vi "StartSequenceAcquisition.vi"(8 "error in (no error)":errorcluster, 10 "DataExchange":T1, 11 "Camera_Prime95B in":refnum<class "Camera_Prime95B.lvclass">) -> (0 "error out":errorcluster, 3 "Camera_Prime95B out":refnum<class "Camera_Prime95B.lvclass">)   [LabVIEW 2020, in "Camera_Prime95B.lvlib" / "Camera_Prime95B.lvclass"]
uses:
  Camera_Prime95B.lvclass
  Hardware Abstraction Layer/Component/Device/Device/DataExchange.ctl
  Controls/AcquisitionParams.ctl
  Controls/Camera Status.ctl
  Camera_Prime95B.lvclass/Camera_Prime95B.ctl
  Hardware Abstraction Layer/Component/Device/Device/DeviceStatus.ctl
  Controls/Wait For Stop Status.ctl
  E:/Development/DevHardSoftware/MicroscopyFramework/Model/Hardware Layer/Real Hardware/Camera_Prime95B/Camera_Prime95B/Dependencies/PVCamNET.dll
  Dependencies/PVCamNET.dll
  Hardware Abstraction Layer/Component/Device/Device/Device.lvlib
  Interface/DataListener/DataListener.lvclass
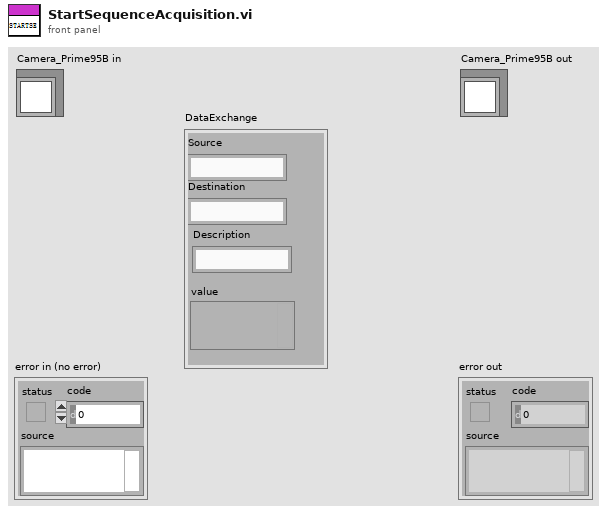
[diagram p1: front panel]
types:
  T1 = typedef "DataListener.lvclass/DataExchange.ctl" = cluster{"Source":string, "Destination":string, "Description":string, "value":variant}
  T2 = typedef "Camera_Prime95B.lvlib/Camera_Prime95B.lvclass/AcquisitionParams.ctl" = cluster{"Acq Mode":T3, "Save Path":path, "Stream Save Path":path, "SingleStack?":bool, "StreamToDisk?":bool, "Alert when finish?":bool}
  T3 = typedef "Camera_Prime95B.lvlib/Camera_Prime95B.lvclass/Camera Status.ctl" = i32
  T4 = typedef "Device.lvlib/DeviceStatus.ctl" = i32
  T5 = typedef "Camera_Prime95B.lvlib/Camera_Prime95B.lvclass/Wait For Stop Status.ctl" = i32
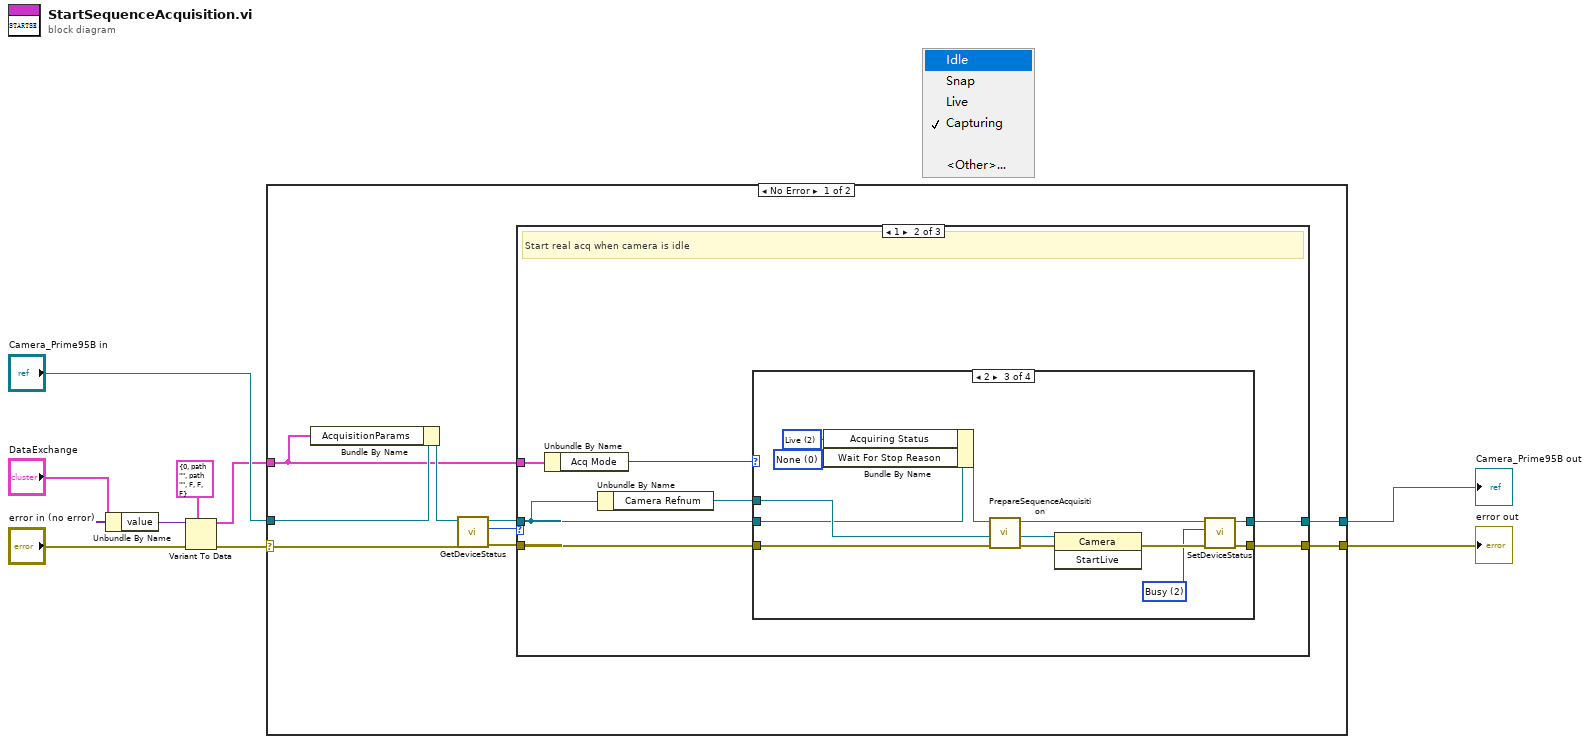
[diagram p0: block diagram]
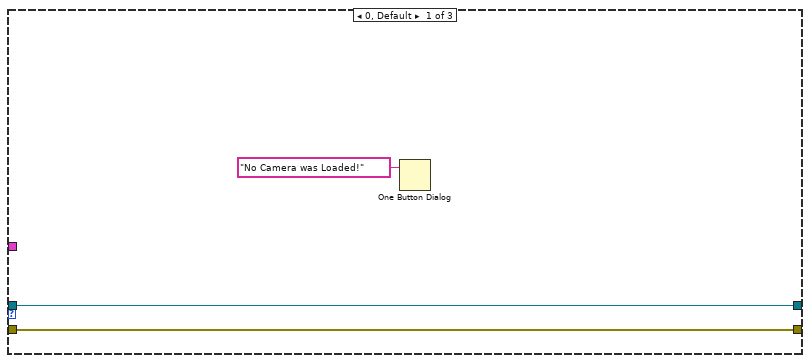
[diagram p2: hidden frame]
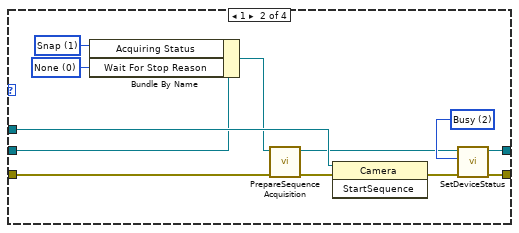
[diagram p4: hidden frame]
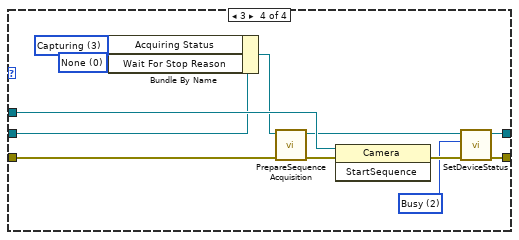
[diagram p5: hidden frame]
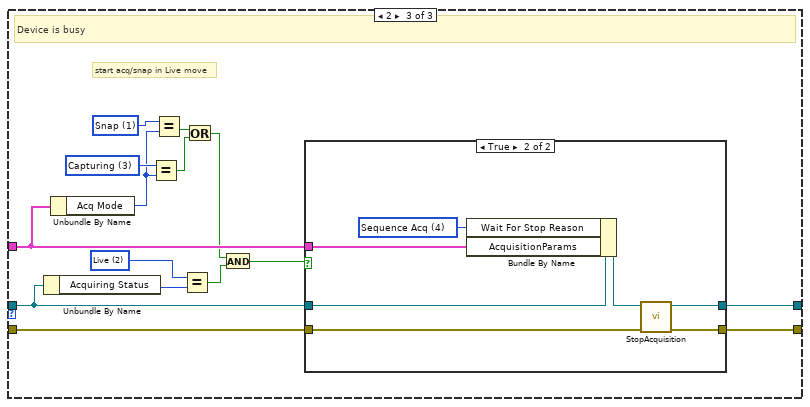
[diagram p6: hidden frame]
diagram:
  n1 = Unbundle By Name("DataExchange") -> ("value"=w5:variant)
  n2 = Variant To Data(error in="error in (no error)", type=T2 {"Acq Mode"=0, "Save Path"=path "", "Stream Save Path"=path "", "SingleStack?"=FALSE, "StreamToDisk?"=FALSE, "Alert when finish?"=FALSE} ("Acquisition Params"), Variant=w5) -> (data=w3:T2, error out=w2:errorcluster)
  n3 = case shown="No Error" w2 {
    selector: w2 -> [w18 w92]
    tunnel: [w15 w92] -> w6
    tunnel: "Camera_Prime95B in" -> [w17 w91]
    tunnel: [w16 w91] -> w7
    tunnel: w3 -> [w10 _]
    frame No Error {
      n4 = Bundle By Name(cluster=w17, "AcquisitionParams"=w10) -> (w11:refnum<class "Camera_Prime95B.lvclass">)
      n5 = call-dynamic "GetDeviceStatus.vi"("error in (no error)"=w18, "Camera_Prime95B in"=w11) -> ("error out"=w13:errorcluster, "Status"=w12:T4, "Camera_Prime95B out"=w14:refnum<class "Camera_Prime95B.lvclass">)  [unwired: 7 in]
      n6 = case shown="1" w12 {
        tunnel: w14 -> [w21 w23 w81]
        tunnel: [w21 w25 w80] -> w16
        tunnel: [w20 w28 w78] -> w15
        tunnel: w13 -> [w20 w26 w79]
        tunnel: w10 -> [_ w24 w77]
        frame 0, Default {
          n7 = One Button Dialog(message="No Camera was Loaded!") -> ()  [unwired: 1 in, 1 out]
        }
        frame 1 {
          # "Start real acq when camera is idle"
          n8 = Unbundle By Name(w24) -> ("Acq Mode"=w22:T3)
          n9 = Unbundle By Name(w23) -> ("Camera Refnum"=w27:refnum<k24>)
          n10 = case shown="2" w22 {
            tunnel: [w29 w39 w51 w63] -> w28
            tunnel: w26 -> [w29 w40 w52 w64]
            tunnel: w27 -> [_ w41 w53 w65]
            tunnel: w23 -> [w30 w32 w48 w57]
            tunnel: [w30 w38 w50 w62] -> w25
            frame 0, Default {
            }
            frame 1 {
              w34 = T3 1 items=["Idle", "Snap", "Live", "Capturing", ""] ("Acquiring Status")
              w35 = T5 0 items=["None", "Set Exposure", "Set Binning", "Set ROI", "Sequence Acq", ""] ("Wait For Stop Reason")
              w37 = T4 2 items=["Offline", "Idle", "Busy"] ("Status")
              n11 = Bundle By Name(cluster=w32, "Acquiring Status"=w34, "Wait For Stop Reason"=w35) -> (w31:refnum<class "Camera_Prime95B.lvclass">)
              n12 = call-dynamic "PrepareSequenceAcquisition.vi"("error in (no error)"=w40, "Camera_Prime95B in"=w31) -> ("error out"=w36:errorcluster, "Camera_Prime95B out"=w33:refnum<class "Camera_Prime95B.lvclass">)  [unwired: 8 in]
              n13 = invoke class="Camera" method="StartSequence"(reference=w41, error in=w36) -> (error out=w42:errorcluster)  [unwired: 1 in, 2 out]
              n14 = call-dynamic "SetDeviceStatus.vi"("error in (no error)"=w42, "Status"=w37, "Device in"=w33) -> ("error out"=w39:errorcluster, "Device out"=w38:refnum<class "Camera_Prime95B.lvclass">)  [unwired: 7 in]
            }
            frame 2 {
              w46 = T5 0 items=["None", "Set Exposure", "Set Binning", "Set ROI", "Sequence Acq", ""] ("Wait For Stop Reason")
              w47 = T3 2 items=["Idle", "Snap", "Live", "Capturing", ""] ("Acquiring Status")
              w49 = T4 2 items=["Offline", "Idle", "Busy"] ("Status")
              n15 = Bundle By Name(cluster=w48, "Acquiring Status"=w47, "Wait For Stop Reason"=w46) -> (w44:refnum<class "Camera_Prime95B.lvclass">)
              n16 = call-dynamic "PrepareSequenceAcquisition.vi"("error in (no error)"=w52, "Camera_Prime95B in"=w44) -> ("error out"=w45:errorcluster, "Camera_Prime95B out"=w43:refnum<class "Camera_Prime95B.lvclass">)  [unwired: 8 in]
              n17 = invoke class="Camera" method="StartLive"(reference=w53, error in=w45) -> (error out=w54:errorcluster)  [unwired: 1 in, 2 out]
              n18 = call-dynamic "SetDeviceStatus.vi"("error in (no error)"=w54, "Status"=w49, "Device in"=w43) -> ("error out"=w51:errorcluster, "Device out"=w50:refnum<class "Camera_Prime95B.lvclass">)  [unwired: 7 in]
            }
            frame 3 {
              w55 = T5 0 items=["None", "Set Exposure", "Set Binning", "Set ROI", "Sequence Acq", ""] ("Wait For Stop Reason")
              w56 = T3 3 items=["Idle", "Snap", "Live", "Capturing", ""] ("Acquiring Status")
              w61 = T4 2 items=["Offline", "Idle", "Busy"] ("Status")
              n19 = Bundle By Name(cluster=w57, "Acquiring Status"=w56, "Wait For Stop Reason"=w55) -> (w58:refnum<class "Camera_Prime95B.lvclass">)
              n20 = call-dynamic "PrepareSequenceAcquisition.vi"("error in (no error)"=w64, "Camera_Prime95B in"=w58) -> ("error out"=w60:errorcluster, "Camera_Prime95B out"=w59:refnum<class "Camera_Prime95B.lvclass">)  [unwired: 8 in]
              n21 = invoke class="Camera" method="StartSequence"(reference=w65, error in=w60) -> (error out=w66:errorcluster)  [unwired: 1 in, 2 out]
              n22 = call-dynamic "SetDeviceStatus.vi"("error in (no error)"=w66, "Status"=w61, "Device in"=w59) -> ("error out"=w63:errorcluster, "Device out"=w62:refnum<class "Camera_Prime95B.lvclass">)  [unwired: 7 in]
            }
          }
        }
        frame 2 {
          w70 = T3 1 items=["Idle", "Snap", "Live", "Capturing", ""] ("x")
          w72 = T3 3 items=["Idle", "Snap", "Live", "Capturing", ""] ("x")
          w73 = T3 2 items=["Idle", "Snap", "Live", "Capturing", ""] ("x")
          # "start acq/snap in Live move"
          # "Device is busy"
          n23 = Unbundle By Name(w81) -> ("Acquiring Status"=w76:T3)
          n24 = Unbundle By Name(w77) -> ("Acq Mode"=w71:T3)
          n25 = Equal?(x=w72, y=w71) -> (x = y?=w69:bool)
          n26 = Equal?(x=w70, y=w71) -> (x = y?=w68:bool)
          n27 = Equal?(x=w73, y=w76) -> (x = y?=w75:bool)
          n28 = Or(x=w68, y=w69) -> (x .or. y?=w67:bool)
          n29 = And(x=w67, y=w75) -> (x .and. y?=w74:bool)
          n30 = case shown="True" w74 {
            tunnel: w79 -> [w82 w90]
            tunnel: [w82 w89] -> w78
            tunnel: w81 -> [w83 w88]
            tunnel: [w83 w86] -> w80
            tunnel: w77 -> [_ w85]
            frame False {
            }
            frame True {
              w84 = T5 4 items=["None", "Set Exposure", "Set Binning", "Set ROI", "Sequence Acq", ""] ("Wait For Stop Reason")
              n31 = Bundle By Name(cluster=w88, "Wait For Stop Reason"=w84, "AcquisitionParams"=w85) -> (w87:refnum<class "Camera_Prime95B.lvclass">)
              n32 = call-dynamic "StopAcquisition.vi"("error in (no error)"=w90, "Camera_Prime95B in"=w87) -> ("error out"=w89:errorcluster, "Camera_Prime95B out"=w86:refnum<class "Camera_Prime95B.lvclass">)  [unwired: 8 in]
            }
          }
        }
      }
    }
    frame Error {
    }
  }
  "error out" <- w6
  "Camera_Prime95B out" <- w7
